vi "GetMemberName.vi"(8 "error in (no error)":errorcluster, 11 "BaseAccessorScripter in":refnum<class "BaseAccessorScripter.lvclass">) -> (0 "error out":errorcluster, 2 "MemberName":string, 3 "BaseAccessorScripter out":refnum<class "BaseAccessorScripter.lvclass">)   [LabVIEW 2021, in "MemberVICreation.lvlib" / "BaseAccessorScripter.lvclass"]
uses:
  <resource>/Framework/Providers/LVClassLibrary/NewAccessors/BaseAccessorScripter/BaseAccessorScripter.lvclass
  <resource>/Framework/Providers/LVClassLibrary/NewAccessors/BaseAccessorScripter/BaseAccessorScripter.lvclass/BaseAccessorScripter.ctl
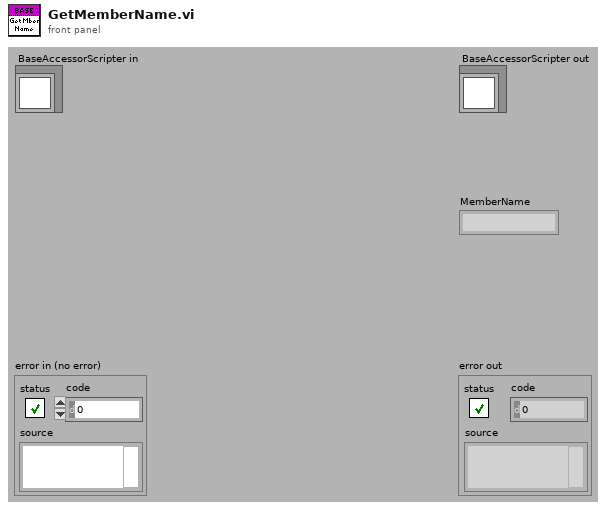
[diagram p1: front panel]
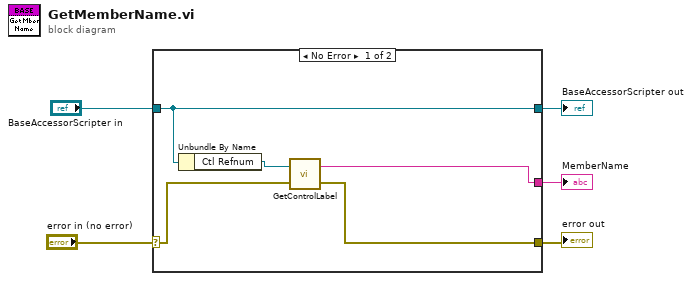
[diagram p0: block diagram]
diagram:
  n1 = case shown="No Error" "error in (no error)" {
    selector: "error in (no error)" -> [w8 w12]
    tunnel: [w6 w12] -> w4
    tunnel: [w10 w11] -> w2
    tunnel: "BaseAccessorScripter in" -> [w10 w11]
    tunnel: [w7 _] -> w1
    frame No Error {
      n2 = Unbundle By Name(w10) -> ("Ctl Refnum"=w9:refnum<vi>)
      n3 = call <resource>:"GetControlLabel.vi"("error IO"=w8, "Ctl Refnum"=w9) -> ("error out"=w6:errorcluster, "Label.Text"=w7:string)
    }
    frame Error {
    }
  }
  "error out" <- w4
  "BaseAccessorScripter out" <- w2
  "MemberName" <- w1
